vi "Evaluate Hall Test 2.vi"(1 "String In":string) -> (0 "Test OK":bool)   [LabVIEW 2023]
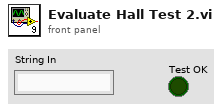
[diagram p1: front panel]
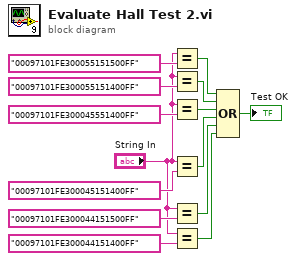
[diagram p0: block diagram]
diagram:
  n1 = Equal?(x="String In", y="00097101FE300055151500FF" ("Self Test BIST")) -> (x = y?=w8:bool)
  n2 = Equal?(x="String In", y="00097101FE300055151400FF") -> (x = y?=w7:bool)
  n3 = Equal?(x="String In", y="00097101FE300045551400FF") -> (x = y?=w6:bool)
  n4 = Equal?(x="String In", y="00097101FE300045151400FF") -> (x = y?=w5:bool)
  n5 = Equal?(x="String In", y="00097101FE300044151500FF") -> (x = y?=w9:bool)
  n6 = Equal?(x="String In", y="00097101FE300044151400FF") -> (x = y?=w1:bool)
  n7 = Compound Arithmetic op=OR(w8, w7, w6, w5, w9, w1) -> (→"Test OK":bool)
